vi "test_cmdbuf.vi"() -> ()   [LabVIEW 2017]
panel:
  out "element":string
  out "data":bool
  out "number (0 to 1)":dbl
  in  "add":bool
  in  "stop":bool
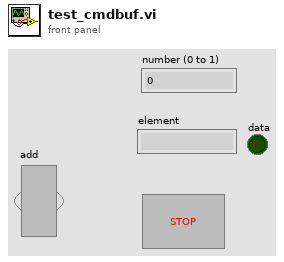
[diagram p1: front panel]
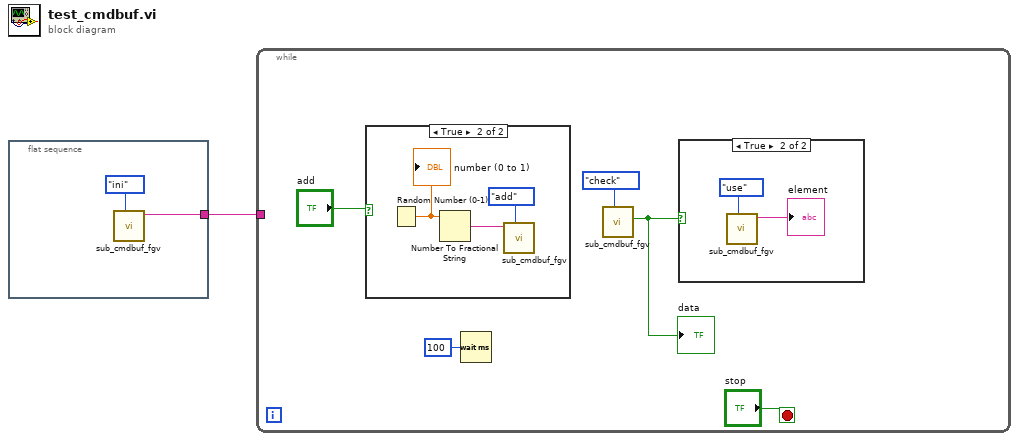
[diagram p0: block diagram]
diagram:
  n1 = flat-sequence {
    tunnel: [w3] -> w1
    frame #0 {
      n2 = call "sub_cmdbuf_fgv.vi"("cmd"=enum16{"ini", "add", "use", "check"}."ini") -> ("element"=w3:string)  [unwired: 9 in, 1 out]
    }
  }
  n3 = while {
    tunnel: w1 -> [_]
    stop <- "stop" stop-if-true
    n4 = case shown="True" "add" {
      frame False {
      }
      frame True {
        n5 = Random Number (0-1)() -> (number: 0 to 1=w13:dbl)
        "number (0 to 1)" <- w13
        n6 = Number To Fractional String(number=w13) -> (F-format string=w12:string)  [unwired: 3 in]
        n7 = call "sub_cmdbuf_fgv.vi"(7:"cmd"=enum16{"ini", "add", "use", "check"}."add" ("cmd"), 11:"cmd"=w12) -> ()  [unwired: 8 in, 2 out]
      }
    }
    n8 = Wait (ms)(milliseconds to wait=u32 100) -> ()  [unwired: 1 out]
    n9 = call "sub_cmdbuf_fgv.vi"("cmd"=enum16{"ini", "add", "use", "check"}."check") -> ("data"=w4:bool)  [unwired: 9 in, 1 out]
    "data" <- w4
    n10 = case shown="True" w4 {
      frame False {
      }
      frame True {
        n11 = call "sub_cmdbuf_fgv.vi"("cmd"=enum16{"ini", "add", "use", "check"}."use") -> ("element"=→"element":string)  [unwired: 9 in, 1 out]
      }
    }
  }
